vi "Generated Descriptors.vi"() -> (3 "Descriptor Strings":string[](array[string]))   [LabVIEW 2025, in "calculator_server.lvlib"]
uses:
  calculator_server.lvlib
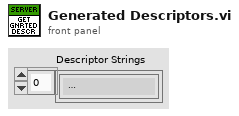
[diagram p1: front panel]
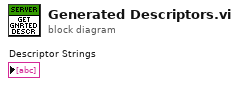
[diagram p0: block diagram]
diagram:
